vi "MPS_Drive_ImonScale.vi"(11 "Drive IMon FFT Mag RMS":dbl) -> (2 "Amps Drive Peak":dbl, 3 "Expected mT Peak":dbl)   [LabVIEW 2021]
uses:
  MPS_global_variables.vi
panel:
  out "Volts per peak amp\nDrive at fDrive":dbl
  out "Drive IMon FFT Mag Peak":dbl
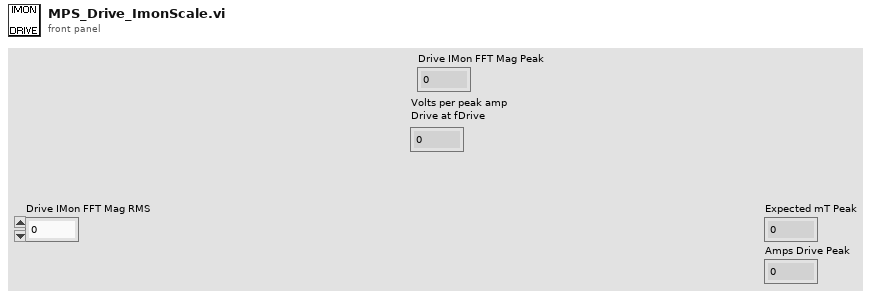
[diagram p1: front panel]
types:
  T1 = cluster{"sample rate":dbl, "Tx freq":dbl, "Tx amp":dbl, "Tx cycles\nSpectroscopy":dbl, "Bias amp":dbl, "Bias freq":dbl, "Receive range":dbl, "Bias Periods\nMagnetometry":dbl, "Tx Freq Division Factor":dbl, "Drive Periods per Bias":dbl, "TX harmonics":dbl[]}
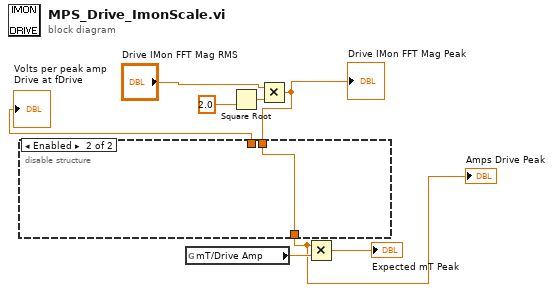
[diagram p0: block diagram]
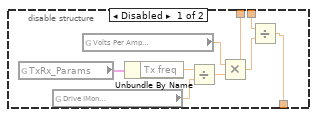
[diagram p2: hidden frame]
diagram:
  n1 = global read "MPS_global_variables.vi" "mT/Drive Amp"() -> (w6:dbl)
  n2 = Square Root(x=2.0) -> (sqrt(x)=w5:dbl)
  n3 = Multiply(x="Drive IMon FFT Mag RMS", y=w5) -> (x*y=w2:dbl)
  "Drive IMon FFT Mag Peak" <- w2
  n4 = disable-structure shown="Enabled" {
    disable-tunnel: [w11 _] -> w7
    disable-tunnel: [w10 w17] -> w1
    disable-tunnel: w2 -> [w9 w17]
    frame Disabled {
      n5 = global read "MPS_global_variables.vi" "TxRx_Params"() -> (w15:T1)
      n6 = global read "MPS_global_variables.vi" "Drive IMon\nRef Freq"() -> (w13:dbl)
      n7 = global read "MPS_global_variables.vi" "Volts Per Amp\nDrive"() -> (w16:dbl)
      n8 = Unbundle By Name(w15) -> ("Tx freq"=w14:dbl)
      n9 = Divide(x=w14, y=w13) -> (x/y=w12:dbl)
      n10 = Multiply(x=w16, y=w12) -> (x*y=w11:dbl)
      n11 = Divide(x=w9, y=w11) -> (x/y=w10:dbl)
    }
    frame Enabled {
    }
  }
  "Volts per peak amp\nDrive at fDrive" <- w7
  "Amps Drive Peak" <- w1
  n12 = Multiply(x=w1, y=w6) -> (x*y=→"Expected mT Peak":dbl)
